vi "Status.Set.vi"(7 "Status Ref":T1, 8 "error in (no error)":errorcluster, 9 "Status":bool) -> (0 "error out":errorcluster)   [LabVIEW 2019, in "Diagnostics Addon Engine.lvlib"]
uses:
  Diagnostics Addon Engine.lvlib
  <vilib>/NI/NIVS Inline Async API/_Data Access Engine/Data Access Engine/Types/Write.DVR.ctl
  <vilib>/NI/NIVS Inline Async API/_Data Access Engine/Access Type Classes/Write/Write.lvclass
  <vilib>/NI/NIVS Inline Async API/_Data Access Engine/Access Type Classes/Write/Write.lvclass/Write.ctl
  <vilib>/NI/NIVS Inline Async API/_Data Access Engine/Data Access Engine/Methods/Write.Data.vi
  <vilib>/NI/NIVS Inline Async API/_Data Access Engine/Access Type Classes/Write/Write.ProcessData.vi
  <vilib>/NI/NIVS Inline Async API/_Data Access Engine/Access Type Classes/Write/Write.Buffer.vi
  <vilib>/NI/NIVS Inline Async API/_Data Access Engine/Access Type Classes/Write/Write.Commit.vi
  <vilib>/NI/NIVS Inline Async API/_Data Access Engine/Data Access Engine/Data Access Engine.lvclass
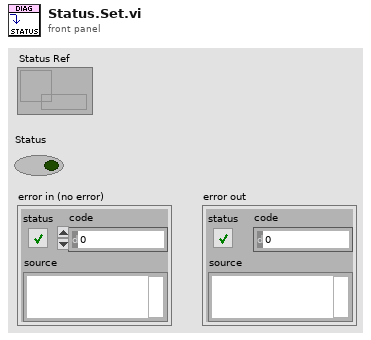
[diagram p1: front panel]
types:
  T1 = typedef "Data Access Engine.lvlib/Data Access Engine.lvclass/Write.DVR.ctl" = refnum<data-value>
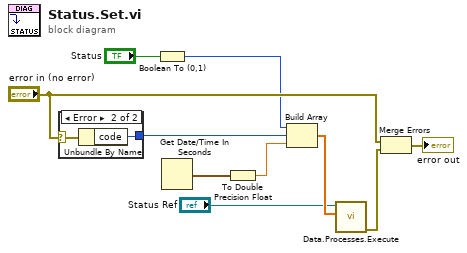
[diagram p0: block diagram]
diagram:
  n1 = case shown="Error" "error in (no error)" {
    selector: "error in (no error)" -> [_ w12]
    tunnel: [_ w11] -> w4
    frame No Error {
    }
    frame Error {
      n2 = Unbundle By Name(w12) -> ("code"=w11:i32)
    }
  }
  n3 = Boolean To (0,1)(Boolean="Status") -> (0, 1=w1:i16)
  n4 = Get Date/Time In Seconds() -> (seconds since 1Jan1904=w5:timestamp)
  n5 = To Double Precision Float(number=w5) -> (double precision float=w3:dbl)
  n6 = Build Array(w1, w4, w3) -> (w9:dbl[])
  n7 = call-poly <vilib>:"Data.Processes.Execute.vi"("Values"=w9, "Ref"="Status Ref") -> ("error out"=w8:errorcluster)  [unwired: 9 in]
  n8 = Merge Errors("error in (no error)", w8) -> (→"error out":errorcluster)
